vi "Open VI.vi"(0 "logic vi path":path, 11 "error in":errorcluster) -> (15 "error out":errorcluster)   [LabVIEW 2021, in "Converter.lvlib"]
uses:
  Converter.lvlib
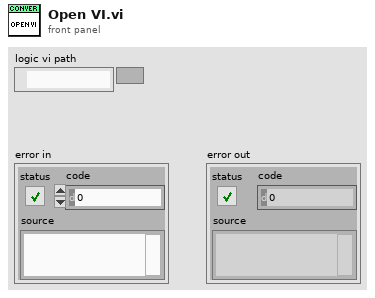
[diagram p1: front panel]
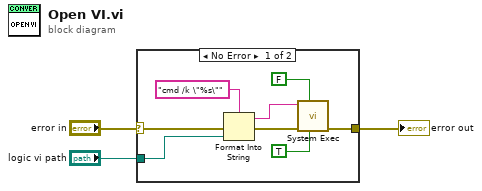
[diagram p0: block diagram]
diagram:
  n1 = case shown="No Error" "error in" {
    selector: "error in" -> [w7 w12]
    tunnel: [w11 w12] -> w3
    tunnel: "logic vi path" -> [w6 _]
    frame No Error {
      n2 = Format Into String(format string="cmd /k \"%s\"", error in=w7, w6) -> (resulting string=w4:string, error out=w10:errorcluster)  [unwired: 1 in]
      n3 = call <vilib>:"System Exec.vi"("run minimized? (F)"=TRUE, "wait until completion? (T)"=FALSE, "error in (no error)"=w10, "command line"=w4) -> ("error out"=w11:errorcluster)  [unwired: 4 in, 3 out]
    }
    frame Error {
    }
  }
  "error out" <- w3
